vi "CaseStructure Get Wire Frame Index.vi"(10 "GObj Refnum":refnum<vi>, 11 "Wire in":refnum<vi>) -> (3 "frame index":i32)   [LabVIEW 2014]
doc: "Returns index of frame which contains specified wire."
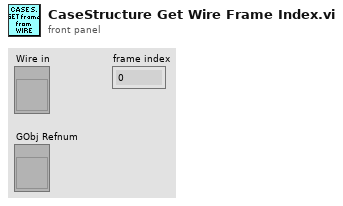
[diagram p1: front panel]
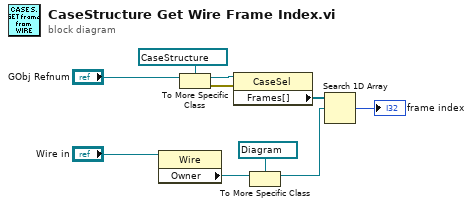
[diagram p0: block diagram]
diagram:
  n1 = property on="Property Node" class="Wire"(reference="Wire in") -> ("Owner"=w10:refnum<vi>)  [unwired: 1 in, 2 out]
  n2 = To More Specific Class(target class=refnum<vi> refnum ("element"), reference="GObj Refnum") -> (specific class reference=w5:refnum<vi>, error out=w6:errorcluster)  [unwired: 1 in]
  n3 = property on="Property Node" class="CaseSel"(reference=w5, error in=w6) -> ("Frames[]"=w7:refnum<vi>[])  [unwired: 2 out]
  n4 = To More Specific Class(target class=refnum<vi> refnum ("element"), reference=w10) -> (specific class reference=w8:refnum<vi>)  [unwired: 1 in, 1 out]
  n5 = Search 1D Array(1D array=w7, element=w8) -> (index of element=→"frame index":i32)  [unwired: 1 in]
